vi "Set Host.vi"(10 "Host":string, 11 "URI in":refnum<class "URI.lvclass">) -> (3 "URI out":refnum<class "URI.lvclass">)   [LabVIEW 2020, in "URI.lvlib" / "URI.lvclass"]
uses:
  URI.lvclass
  URI.lvclass/URI.ctl
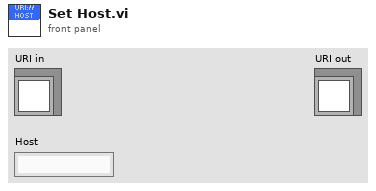
[diagram p1: front panel]
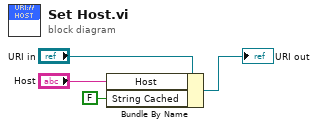
[diagram p0: block diagram]
diagram:
  n1 = Bundle By Name(cluster="URI in", "Host"="Host", "String Cached"=FALSE) -> (→"URI out":refnum<class "URI.lvclass">)
